vi "Delete Active DUT Band.vi"(8 "error in (no error)":errorcluster, 11 "VISA resource name":refnum<visa-resource-name>) -> (0 "error out":errorcluster, 3 "VISA resource name out":refnum<visa-resource-name>)   [LabVIEW 2015, in "Rohde&Schwarz CMXP Base.lvlib"]
doc: "Removes frequency bands from all antenna connectors of the active DUT.\n\nYou can remove several bands with a single command. Specify the technology and the band number for each band.\n\nAttribute:\n-\n\nRemote-control command:\nREMove:DUT:BAND"
uses:
  <instrlib>/Rohde&Schwarz CMXP Base/Rohde&Schwarz CMXP Base.lvlib
  <instrlib>/Rohde&Schwarz CMXP Base/Private/rsidr_core.llb/rsidr_core.lvlib
panel:
  in  "Bands":cluster{"Type (LTE)":i32, "Band Number":i32}[](array[cluster]) {"Type (LTE)" items=["LTE", "New Radio", "WLAN"]}
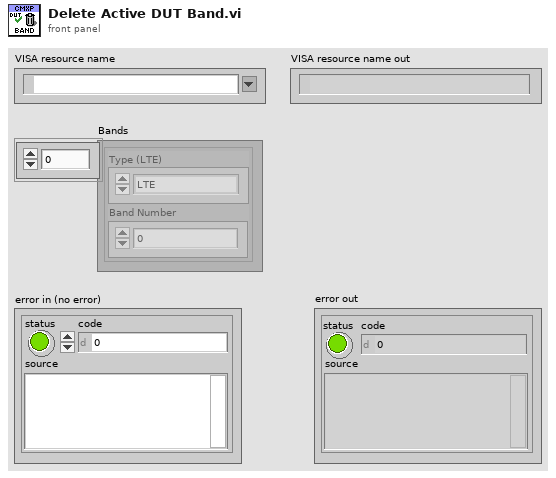
[diagram p1: front panel]
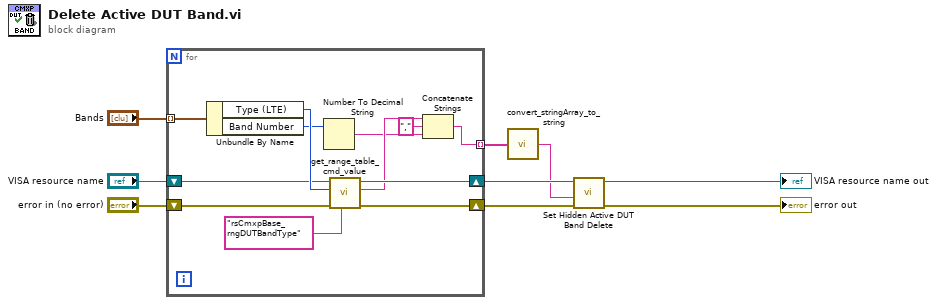
[diagram p0: block diagram]
diagram:
  n1 = for {
    tunnel: "Bands" -> [w21] mode=indexing
    tunnel: [w16] -> w7 mode=indexing
    shift-right: [w18] -> w2
    shift-left: "VISA resource name" -> [w10]
    shift-right: [w17] -> w3
    shift-left: "error in (no error)" -> [w11]
    n2 = Unbundle By Name(w21) -> ("Type (LTE)"=w20:i32, "Band Number"=w13:i32)
    n3 = Number To Decimal String(number=w13) -> (decimal integer string=w12:string)  [unwired: 1 in]
    n4 = call <instrlib>:"get_range_table_cmd_value.vi"("Range Table ID in"="rsCmxpBase_rngDUTBandType", "error in"=w11, "Input Int32 value"=w20, "VISA resource name"=w10) -> ("error out"=w17:errorcluster, "Cmd value out"=w15:string, "VISA resource name out"=w18:refnum<visa-resource-name>)  [unwired: 5 in]
    n5 = Concatenate Strings(w15, "," ("string"), w12) -> (w16:string)
  }
  n6 = call <instrlib>:"convert_stringArray_to_string.vi"("string array in"=w7) -> ("string out"=w1:string)  [unwired: 4 in]
  n7 = call "Set Hidden Active DUT Band Delete"("error in (no error)"=w3, "Hidden Active DUT Band Delete ()"=w1, "instrument handle"=w2) -> ("error out"=→"error out":errorcluster, "instrument handle out"=→"VISA resource name out":refnum<visa-resource-name>)  [unwired: 7 in]
